vi "GetTimestamp.vi"(8 "error in (no error)":errorcluster) -> (0 "error out":errorcluster, 3 "date/time string":string)   [LabVIEW 2016]
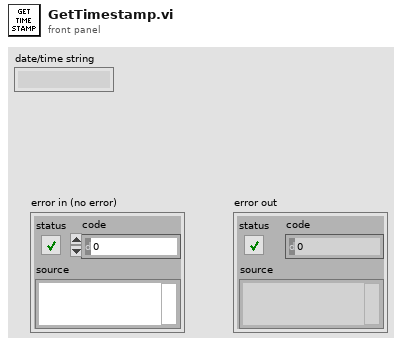
[diagram p1: front panel]
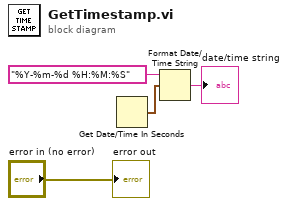
[diagram p0: block diagram]
diagram:
  n1 = Get Date/Time In Seconds() -> (seconds since 1Jan1904=w4:timestamp)
  n2 = Format Date/Time String(time format string (%c)="%Y-%m-%d %H:%M:%S", seconds (now)=w4) -> (date/time string=→"date/time string":string)  [unwired: 1 in]
  "error out" <- "error in (no error)"
